vi "Get ProjectItem Descendants (with Pattern).vi"(7 "Type":string, 8 "error in (no error)":errorcluster, 10 "Pattern":string, 11 "ProjectItem in":refnum<vi>) -> (0 "error out":errorcluster, 2 "ProjectItem descendents":refnum<vi>[](array[refnum]), 3 "ProjectItem out":refnum<vi>)   [LabVIEW 2019, in "gRPC Template Creation Utility.lvlib"]
uses:
  gRPC Template Creation Utility.lvlib
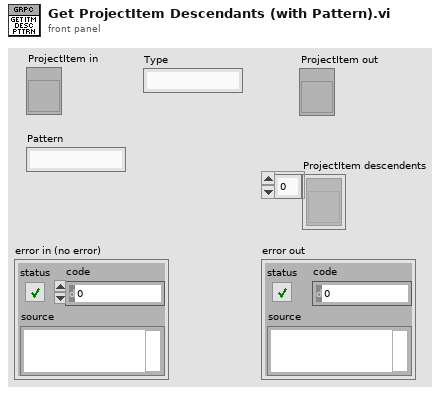
[diagram p1: front panel]
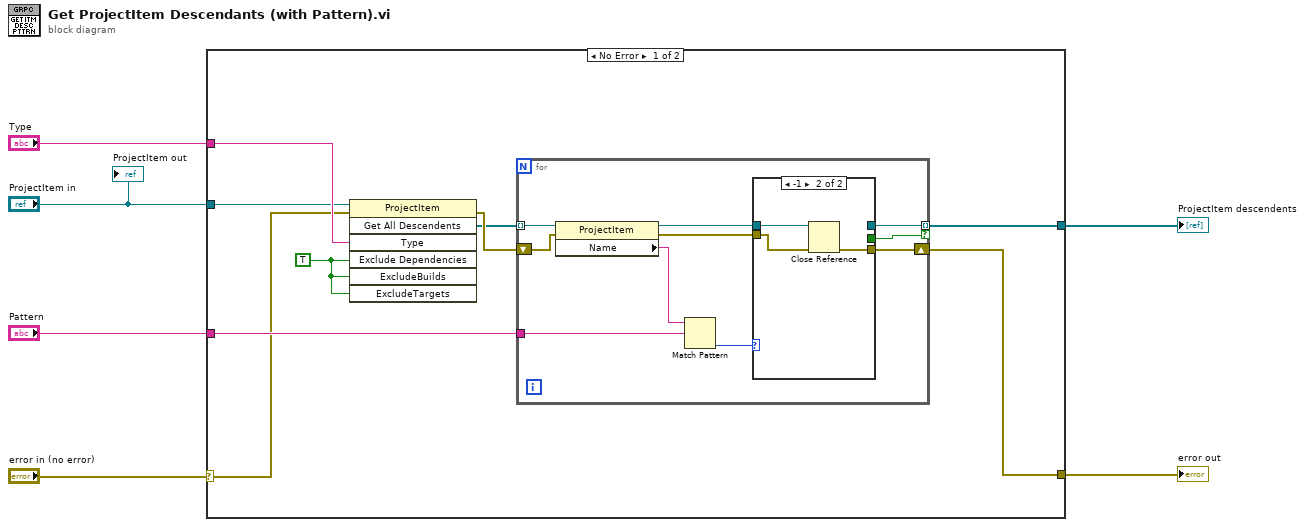
[diagram p0: block diagram]
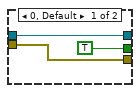
[diagram p2: hidden frame]
diagram:
  n1 = case shown="No Error" "error in (no error)" {
    selector: "error in (no error)" -> [w9 w32]
    tunnel: "Pattern" -> [w14 _]
    tunnel: "Type" -> [w11 _]
    tunnel: "ProjectItem in" -> [w10 _]
    tunnel: [w8 w32] -> w2
    tunnel: [w7 _] -> w1
    frame No Error {
      w12 = TRUE ("ExcludeDependencies")
      n2 = invoke class="ProjectItem" method="Get All Descendents"(reference=w10, error in=w9, "Type"=w11, "Exclude Dependencies"=w12, "ExcludeBuilds"=w12, "ExcludeTargets"=w12) -> (error out=w15:errorcluster, "All Descendents"=w13:refnum<vi>[])  [unwired: 1 in, 5 out]
      n3 = for {
        tunnel: w13 -> [w25] mode=indexing
        tunnel: w14 -> [w23]
        tunnel: [w18] -> w7 mode=indexing if=w16
        shift-right: [w17] -> w8
        shift-left: w15 -> [w22]
        n4 = property class="ProjectItem"(reference=w25, error in=w22) -> (reference out=w20:refnum<vi>, error out=w19:errorcluster, "Name"=w24:string)
        n5 = Match Pattern(string=w24, regular expression=w23) -> (offset past match=w21:i32)  [unwired: 1 in, 3 out]
        n6 = case shown="-1" w21 {
          tunnel: w20 -> [w28 w30]
          tunnel: w19 -> [w26 w31]
          tunnel: [w26 w29] -> w17
          tunnel: [w28 _] -> w18
          tunnel: [TRUE _] -> w16
          frame 0, Default {
          }
          frame -1 {
            n7 = Close Reference(reference=w30, error in (no error)=w31) -> (error out=w29:errorcluster)
          }
        }
      }
    }
    frame Error {
    }
  }
  "error out" <- w2
  "ProjectItem descendents" <- w1
  "ProjectItem out" <- "ProjectItem in"
